vi "interpolate.vi"() -> ()   [LabVIEW 2014]
panel:
  in  "value in 2":dbl=5.0
  out "value map 2":dbl=2.5
  out "fractional index or x 3":dbl=0.5
  out "value map":dbl=2.5
  in  "value in":dbl=5.0
  out "fractional index or x 2":dbl=0.9
  in  "threshold y":dbl=9.0
  in  "fractional index or x":dbl=0.9
  out "y value":dbl=4.5
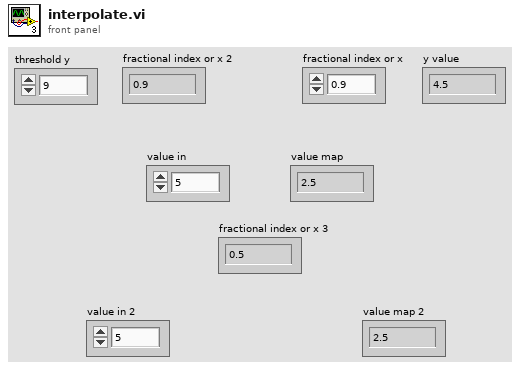
[diagram p1: front panel]
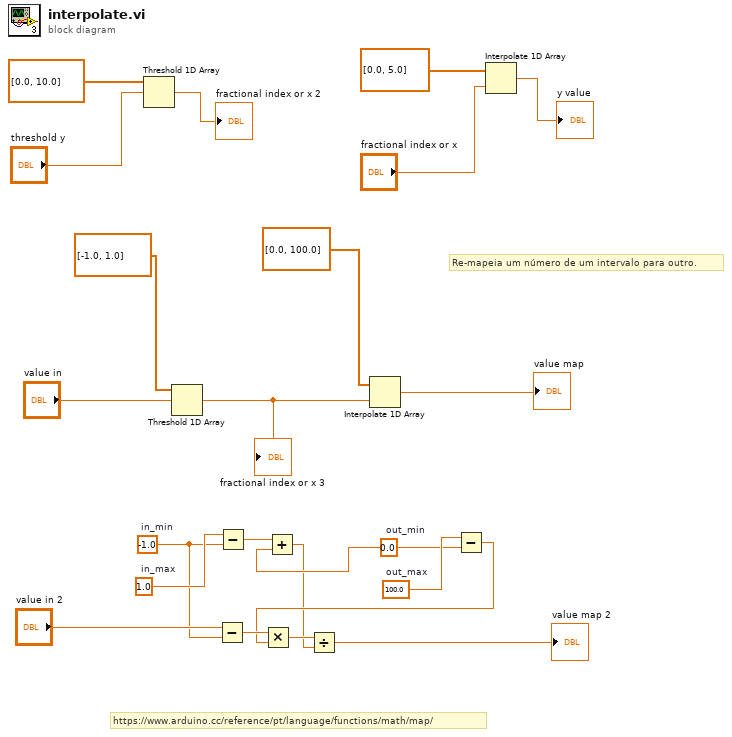
[diagram p0: block diagram]
diagram:
  w10 = 100.0  # out_max
  w3 = 0.0  # out_min
  w7 = 1.0  # in_max
  w4 = -1.0  # in_min
  # "https://www.arduino.cc/reference/pt/language/functions/math/map/"
  # "Re-mapeia um número de um intervalo para outro."
  n1 = Threshold 1D Array(2:"threshold y", 3:dbl[] [0.0, 10.0] ("array of numbers or points")) -> (0:→"fractional index or x 2":dbl)  [unwired: 1 in]
  n2 = Threshold 1D Array(2:"value in", 3:dbl[] [-1.0, 1.0] ("array of numbers or points")) -> (0:w16:dbl)  [unwired: 1 in]
  "fractional index or x 3" <- w16
  n3 = Subtract(x="value in 2", y=w4) -> (x-y=w9:dbl)
  n4 = Subtract(x=w7, y=w4) -> (x-y=w5:dbl)
  n5 = Add(x=w5, y=w3) -> (x+y=w2:dbl)
  n6 = Interpolate 1D Array(1:w16, 2:dbl[] [0.0, 100.0] ("array of numbers or points")) -> (0:→"value map":dbl)
  n7 = Subtract(x=w10, y=w3) -> (x-y=w8:dbl)
  n8 = Multiply(x=w9, y=w8) -> (x*y=w6:dbl)
  n9 = Divide(x=w6, y=w2) -> (x/y=→"value map 2":dbl)
  n10 = Interpolate 1D Array(1:"fractional index or x", 2:dbl[] [0.0, 5.0] ("array of numbers or points")) -> (0:→"y value":dbl)
